vi "Baseband Transmission-Simple - Template.vi"() -> ()   [LabVIEW 2013]
uses:
  <vilib>/Analysis/2dsp.llb/1D Convolution (DBL).vi
  <vilib>/Analysis/2dsp.llb/Decimate (single shot, DBL).vi
  <vilib>/Analysis/2dsp.llb/Upsample (DBL).vi
  <vilib>/Analysis/NI_AALPro.lvlib
  <vilib>/Analysis/NI_AALBase.lvlib
panel:
  in  "Sinc Samples":i32=65
  out "Recovered Bits":i32[](array[numeric])
  in  "stop":bool
  in  "UpSample Factor":i32(slide)=74 scale=1.0..100.0
  out "Symbol":dbl[](array[numeric])
  in  "Bit":i32[](array[numeric])=[0, 0, 0, 1, 0, 1, 1, 1, 0, 0]
  in  "Pulse Shaping Function":enum16{"Triangle", "Sinc", "Rcosine"}(ring)=enum."Sinc"
  out "Pulse Shaping":dbl[][](graph)
  out "Baseband":dbl[](graph)
  # "Baseband Transmission"
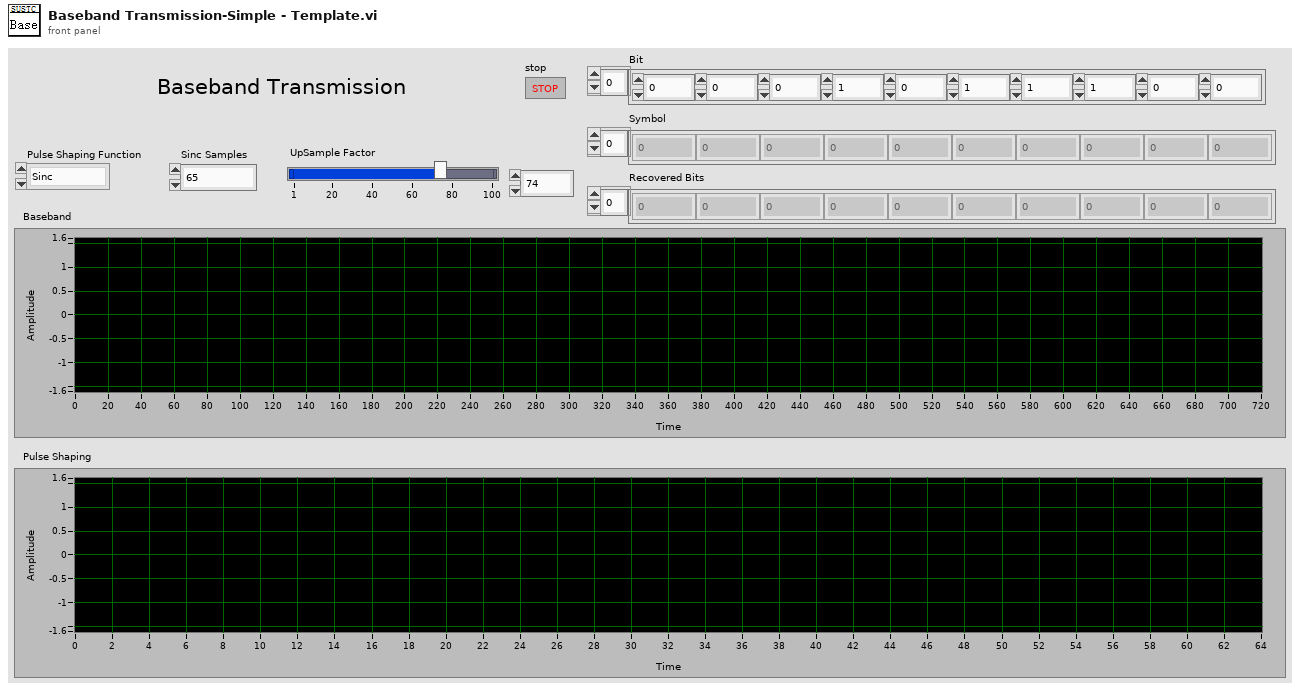
[diagram p1: front panel]
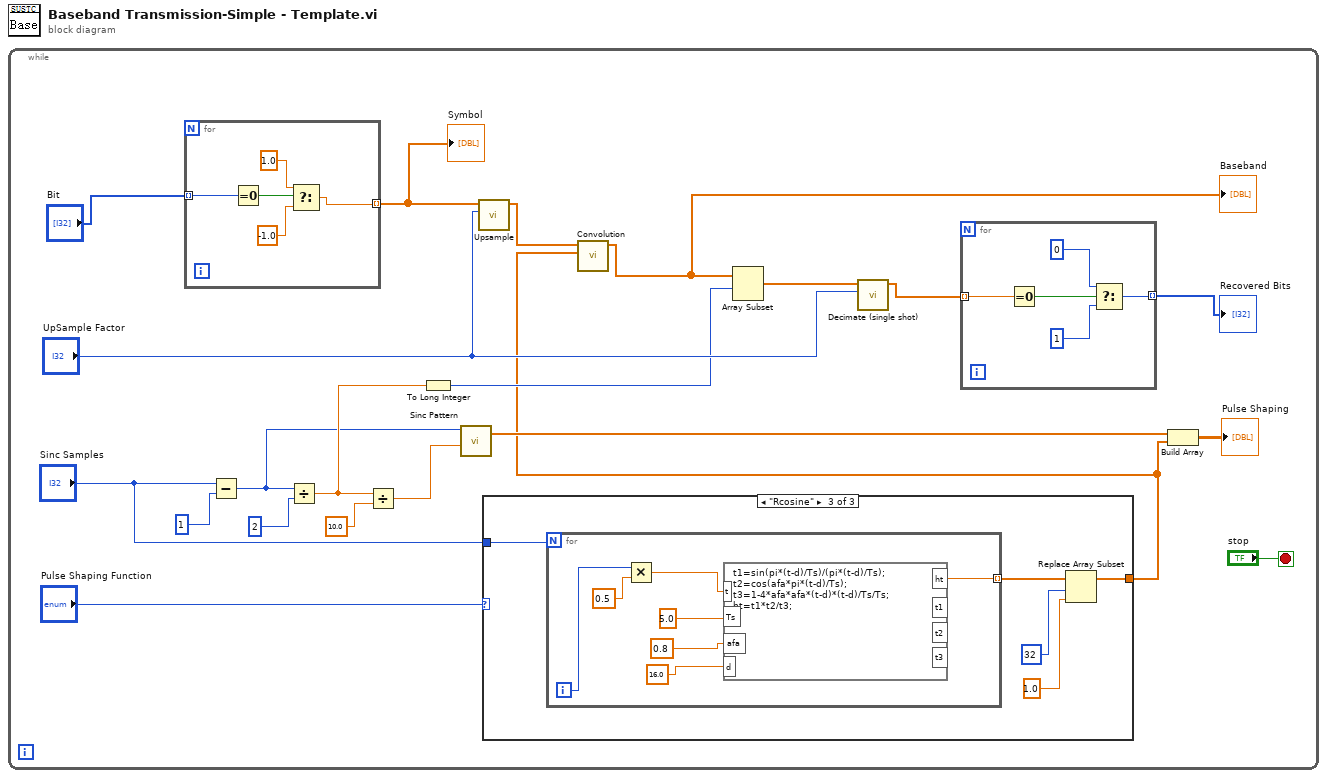
[diagram p0: block diagram]
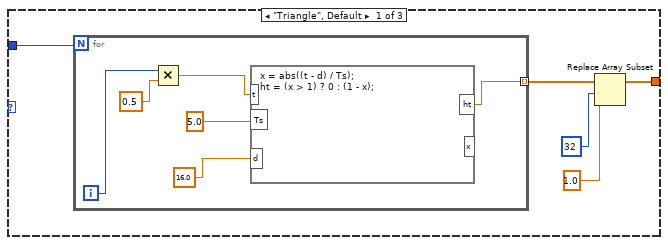
[diagram p2: hidden frame]
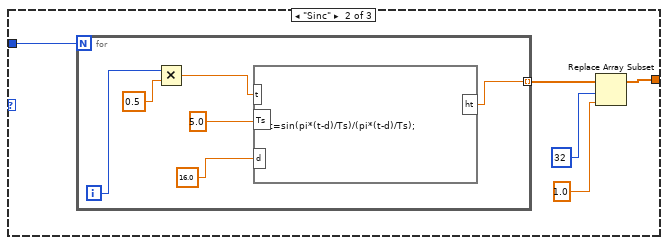
[diagram p3: hidden frame]
diagram:
  n1 = while {
    stop <- "stop" stop-if-true
    n2 = for {
      tunnel: "Bit" -> [w65] mode=indexing
      tunnel: [w61] -> w19 mode=indexing
      n3 = Equal To 0?(x=w65) -> (x = 0?=w64:bool)
      n4 = Select(t=1.0, s=w64, f=-1.0) -> (s? t:f=w61:dbl)
    }
    "Symbol" <- w19
    n5 = Subtract(x="Sinc Samples", y=1) -> (x-y=w12:i32)
    n6 = Divide(x=w12, y=2) -> (x/y=w13:dbl)
    n7 = Divide(x=w13, y=10.0) -> (x/y=w11:dbl)
    n8 = To Long Integer(number=w13) -> (32bit integer=w5:i32)
    n9 = call <vilib>:"Sinc Pattern.vi"("delay"=w11, "samples"=w12) -> ("Sinc Pattern"=w4:dbl[])  [unwired: 2 in, 1 out]
    n10 = call-poly <vilib>:"Upsample.vi"("upsampling factor"="UpSample Factor", "X"=w19) -> ("Upsampled Array"=w18:dbl[])  [unwired: 8 in, 1 out]
    n11 = case shown="\"Rcosine\"" "Pulse Shaping Function" {
      tunnel: [w27 w40 w50] -> w2
      tunnel: "Sinc Samples" -> [w28 w39 w49]
      frame "Triangle", Default {
        n12 = for {
          N: w28 -> [_]
          tunnel: [w35] -> w29 mode=indexing
          i -> [w37]
          n13 = Multiply(x=w37, y=0.5) -> (x*y=w34:dbl)
          n14 = formula code="x = abs((t - d) / Ts);\nht = (x > 1) ? 0 : (1 - x);"("t"=w34, "Ts"=5.0, "d"=16.0) -> ("ht"=w35:dbl)  [unwired: 1 out]
        }
        n15 = Replace Array Subset(array=w29, new element=1.0, index=32) -> (w27:dbl[])
      }
      frame "Sinc" {
        n16 = for {
          N: w39 -> [_]
          tunnel: [w46] -> w38 mode=indexing
          i -> [w48]
          n17 = Multiply(x=w48, y=0.5) -> (x*y=w45:dbl)
          n18 = formula code="ht=sin(pi*(t-d)/Ts)/(pi*(t-d)/Ts);"("t"=w45, "Ts"=5.0, "d"=16.0) -> ("ht"=w46:dbl)
        }
        n19 = Replace Array Subset(array=w38, new element=1.0, index=32) -> (w40:dbl[])
      }
      frame "Rcosine" {
        n20 = for {
          N: w49 -> [_]
          tunnel: [w58] -> w51 mode=indexing
          i -> [w60]
          n21 = Multiply(x=w60, y=0.5) -> (x*y=w57:dbl)
          n22 = formula code="t1=sin(pi*(t-d)/Ts)/(pi*(t-d)/Ts);\nt2=cos(afa*pi*(t-d)/Ts);\nt3=1-4*afa*afa*(t-d)*(t-d)/Ts/Ts;\nht=t1*t2/t3;"("t"=w57, "Ts"=5.0, "d"=16.0, "afa"=0.8) -> ("ht"=w58:dbl)  [unwired: 3 out]
        }
        n23 = Replace Array Subset(array=w51, new element=1.0, index=32) -> (w50:dbl[])
      }
    }
    n24 = call-poly <vilib>:"Convolution.vi"("Y"=w2, "X"=w18) -> ("X * Y"=w6:dbl[])  [unwired: 8 in, 1 out]
    "Baseband" <- w6
    n25 = Array Subset(array=w6, index=w5) -> (w10:dbl[])  [unwired: 1 in]
    n26 = call-poly <vilib>:"Decimate (single shot).vi"("decimating factor"="UpSample Factor", "X"=w10) -> ("Decimated Array"=w8:dbl[])  [unwired: 8 in, 1 out]
    n27 = for {
      tunnel: w8 -> [w26] mode=indexing
      tunnel: [w22] -> w7 mode=indexing
      n28 = Equal To 0?(x=w26) -> (x = 0?=w25:bool)
      n29 = Select(t=0, s=w25, f=1) -> (s? t:f=w22:i32)
    }
    "Recovered Bits" <- w7
    n30 = Build Array(w4, w2) -> (→"Pulse Shaping":dbl[][])
  }
